vi "medicaoIXV.vi"() -> ()   [LabVIEW 2012]
uses:
  <vilib>/Utility/file.llb/Write To Spreadsheet File (string).vi
  <vilib>/Utility/file.llb/Write To Spreadsheet File (DBL).vi
  <instrlib>/Agilent 6XXX Series/Agilent 6XXX Series.lvlib
panel:
  out "Ponto Atual":i32
  out "Corrente Atual":dbl
  out "Tensao Atual":dbl
  in  "CorrenteGraph":dbl
  in  "error in (no error)":errorcluster
  out "error out":errorcluster
  out "output voltage":dbl
  in  "delay(s)":dbl
  out "IXV":cluster{"Y":dbl[], "Y":dbl[]}[](graph)
  in  "TensaoGraph":dbl
  in  "Local":path
  in  "Start":bool
  in  "Nome da célula":string
  in  "Tensão máxima":dbl
  in  "Pontos":dbl
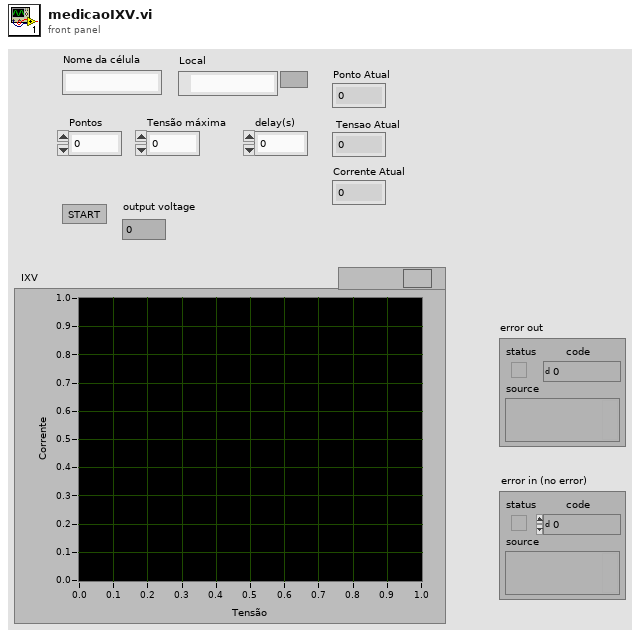
[diagram p1: front panel]
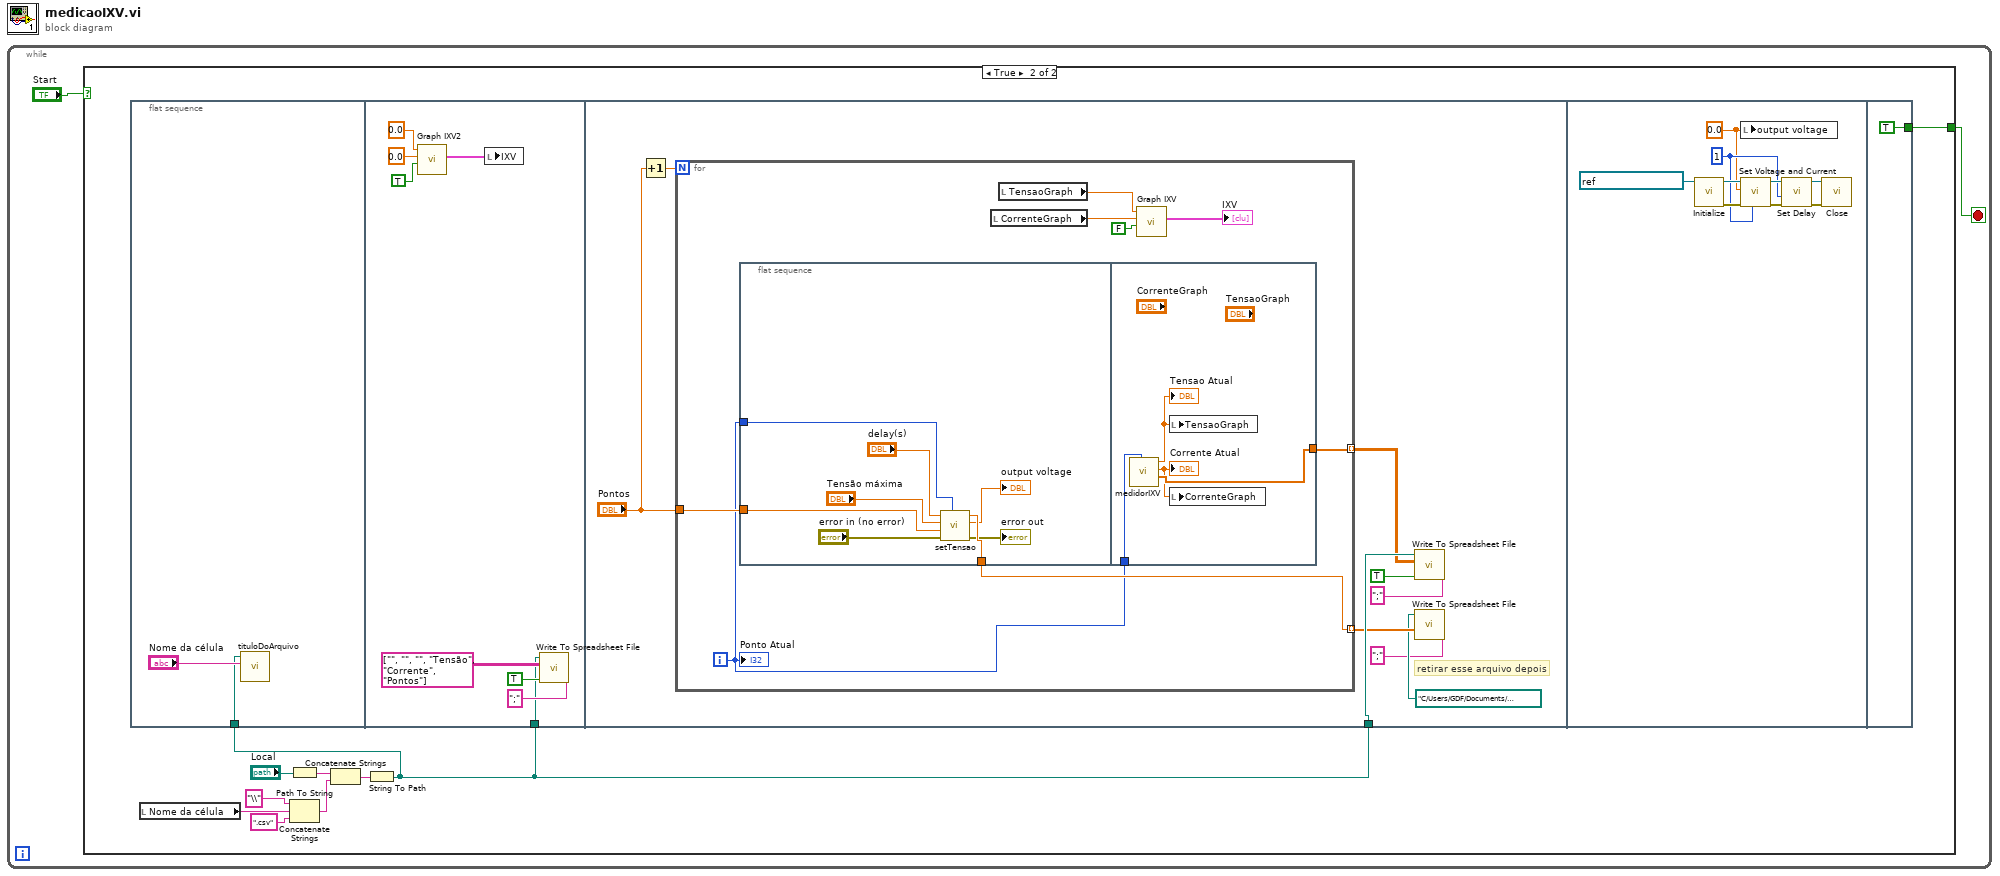
[diagram p0: block diagram]
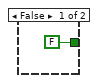
[diagram p2: hidden frame]
diagram:
  n1 = while {
    stop <- w1 stop-if-true
    n2 = case shown="True" "Start" {
      tunnel: [FALSE w6] -> w1
      frame False {
      }
      frame True {
        n3 = flat-sequence {
          tunnel: w4 -> [w13]
          tunnel: w4 -> [w19]
          tunnel: w4 -> [w29]
          tunnel: [TRUE] -> w6
          frame #0 {
            n4 = call "tituloDoArquivo.vi"("Nome da célula"="Nome da célula", "Path"=w13) -> ()  [unwired: 10 in]
          }
          frame #1 {
            n5 = call "Graph IXV2"("Reset"=TRUE, "Y Input"=0.0, "X Input"=0.0) -> ("XY Graph"=w15:cluster{"Y":dbl[], "Y":dbl[]}[])  [unwired: 2 in, 6 out]
            n6 = local write "IXV"(w15) -> ()
            n7 = call-poly <vilib>:"Write To Spreadsheet File.vi"("delimiter (\\t)"=";" ("delimiter (\\t)"), "append to file? (new file:F)"=TRUE, "2D data"=string[][] [["", "", ""], ["Tensão", "Corrente", "Pontos"]], "file path (dialog if empty)"=w19) -> ()  [unwired: 4 in, 1 out]
          }
          frame #2 {
            # "retirar esse arquivo depois"
            n8 = Increment(x="Pontos") -> (x+1=w24:dbl)
            n9 = for {
              N: w24 -> [_]
              tunnel: [w39] -> w28 mode=indexing
              tunnel: [w38] -> w27 mode=indexing
              tunnel: "Pontos" -> [w37]
              i -> [w36]
              n10 = flat-sequence {
                tunnel: w37 -> [w43]
                tunnel: [w42] -> w38
                tunnel: w36 -> [w44]
                tunnel: [w51] -> w39
                tunnel: w36 -> [w50]
                frame #0 {
                  n11 = call "setTensao.vi"("Numeric"=w44, "error in (no error)"="error in (no error)", "Pontos"=w43, "Tensão máxima"="Tensão máxima", "delay(s)"="delay(s)") -> ("error out"=→"error out":errorcluster, "output voltage"=→"output voltage":dbl, "output voltage 2"=w42:dbl)  [unwired: 4 in]
                }
                frame #1 {
                  n12 = call "medidorIXV.vi"("Numeric"=w50) -> ("Array"=w51:dbl[], "Corrente Atual"=w48:dbl, "Tensao Atual"=w49:dbl)  [unwired: 8 in]
                  "Corrente Atual" <- w48
                  "Tensao Atual" <- w49
                  n13 = local write "TensaoGraph"(w49) -> ()
                  n14 = local write "CorrenteGraph"(w48) -> ()
                }
              }
              n15 = local read "CorrenteGraph"() -> (w35:dbl)
              n16 = local read "TensaoGraph"() -> (w34:dbl)
              n17 = call "Graph IXV"("Reset"=FALSE, "Y Input"=w35, "X Input"=w34) -> ("XY Graph"=→"IXV":cluster{"Y":dbl[], "Y":dbl[]}[])  [unwired: 2 in, 6 out]
              "Ponto Atual" <- w36
            }
            n18 = call-poly <vilib>:"Write To Spreadsheet File.vi"("delimiter (\\t)"=";" ("delimiter (\\t)"), "append to file? (new file:F)"=TRUE, "2D data"=w28, "file path (dialog if empty)"=w29) -> ()  [unwired: 4 in, 1 out]
            n19 = call-poly <vilib>:"Write To Spreadsheet File.vi"("delimiter (\\t)"=";" ("delimiter (\\t)"), "1D data"=w27, "file path (dialog if empty)"=path "C:/Users/GDF/Documents/ProgramasDeAprendizado/Yan/LabView Aprendizado/2017-03-09 medicaoIXV(teste com dados aleatorios)/testes") -> ()  [unwired: 5 in, 1 out]
          }
          frame #3 {
            w52 = 0.0 ("voltage (0 V)")
            w55 = u8 1 ("channel (1)")
            n20 = call <instrlib>:"Initialize.vi"("VISA resource name"=refnum<visa-resource-name> "GPIB0::5::INSTR") -> ("error out"=w57:errorcluster, "VISA resource name out"=w56:refnum<visa-resource-name>)  [unwired: 9 in]
            n21 = local write "output voltage"(w52) -> ()
            n22 = call <instrlib>:"Set Voltage and Current.vi"("channel (1)"=w55, "error in (no error)"=w57, "voltage (0 V)"=w52, "VISA resource name"=w56) -> ("error out"=w58:errorcluster, "VISA resource name out"=w59:refnum<visa-resource-name>)  [unwired: 6 in]
            n23 = call <instrlib>:"Set Delay.vi"("error in (no error)"=w58, "channel (1)"=w55, "VISA resource name"=w59) -> ("error out"=w53:errorcluster, "VISA resource name out"=w54:refnum<visa-resource-name>)  [unwired: 7 in]
            n24 = call <instrlib>:"Close.vi"("error in (no error)"=w53, "VISA resource name"=w54) -> ()  [unwired: 9 in, 1 out]
          }
          frame #4 {
          }
        }
        n25 = local read "Nome da célula"() -> (w7:string)
        n26 = Path To String(path="Local") -> (string=w11:string)
        n27 = Concatenate Strings("\\", w7, ".csv") -> (w12:string)
        n28 = Concatenate Strings(w11, w12) -> (w10:string)
        n29 = String To Path(string=w10) -> (path=w4:path)
      }
    }
  }
